vi "svx_Build Orbit and Timebase Data (Unfiltered).vi"(4 "pair index":cluster{"index 1":i32, "index 2":i32}[](array[cluster]), 6 "channel properties":T5[](array[typedef]) {"probe angle [deg]" max=360; "direction" items=["CCW", "CW"]}, 8 "error in (no error)":errorcluster, 9 "interpolated pulse positions[s]":dbl[](array[numeric]) format="%.2f", 10 "even-angle channel info":T1[](array[typedef]) {"channel info"."pregain" format="%.2f"; "channel info"."weighting filter" items=["Linear", "A-weighting", "B-weighting", "C-weighting", "ITU-R 468-4", "Dolby", "CCITT", "C-message", "Wb", "Wc", "Wd", "We", "Wf", "Wh", "Wj", "Wk", "Wm", "AES17 20 kHz lowpass", "AES17 40 kHz lowpass", "AES17 20 kHz highpass", "AES17 40 kHz highpass"]; "channel info"."dB reference" format="%^.1e"; "channel info"."engineering units" items=["custom..."=0, "V"=1, "A"=21, "C"=30, "pC"=31, "s"=32, "-"=29, "Pa"=2, "N"=20, "g"=3, "m/s^2"=4, "m/s"=5, "m"=6, "mm/s"=12, "mm"=13, "micron/s"=14, "micron"=15, "in/s^2"=7, "in/s"=8, "in"=9, "mil/s"=10, "mil"=11, "rad/s^2"=16, "rad/s"=17, "rad"=18, "deg/s^2"=26, "deg/s"=27, "deg"=28, "RPM"=22, "cycle/s^2"=23, "Hz"=24, "cycle"=25, "strain"=19]; "channel info"."sensor sensitivity" format="%#_5f"}, 11 "resampled signal out":cluster{dbl[], dbl}[](array[cluster])) -> (0 "error out":errorcluster, 3 "orbit/timebase plot":T6(array[cluster]))   [LabVIEW 2017]
uses:
  <vilib>/addons/Sound and Vibration/Order Analysis/Data Presentation/SubVIs/OAT MCM Channel Property.ctl
  <vilib>/addons/_NISVFA/_Shared subVIs/Controls/svc_Resampled Channel Info.ctl
  <vilib>/addons/_NISVFA/_Shared subVIs/Controls/svc_Channel Info.ctl
  <vilib>/addons/_NISVFA/_Shared subVIs/Controls/svc_Engineering Units Text Ring.ctl
  <vilib>/addons/_NISVFA/_Shared subVIs/Controls/svc_Weighting Filter Text Ring.ctl
  <vilib>/addons/Sound and Vibration/Order Analysis/Misc/SVMS Attribute.ctl
  <vilib>/addons/_NISVFA/_Shared subVIs/Controls/NI Channel Properties.ctl
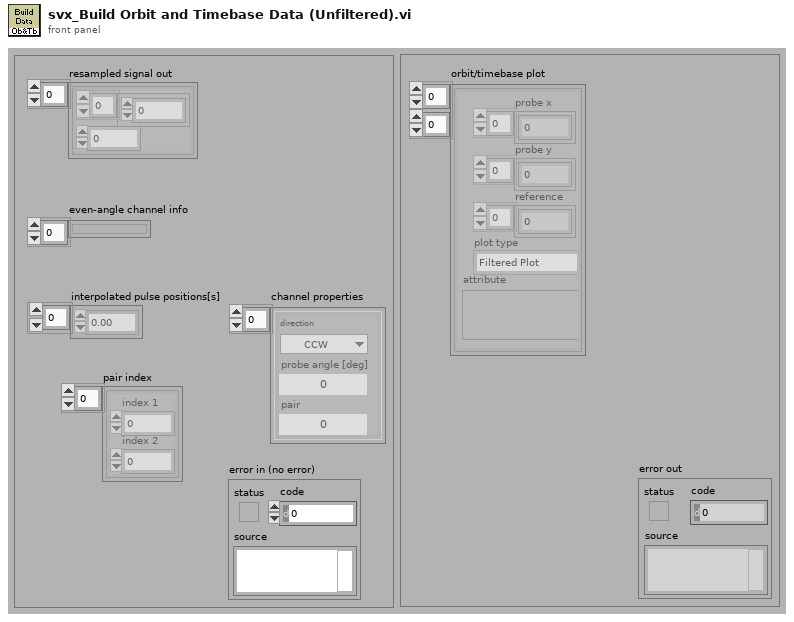
[diagram p1: front panel]
types:
  T1 = typedef "svc_Resampled Channel Info.ctl" = cluster{"channel name":string, "description":string, " channel info":T2}
  T2 = typedef "svc_Channel Info.ctl" = cluster{"sensor sensitivity":dbl, "engineering units":T3, "dB reference":dbl, "custom label":string, "weighting filter":T4, "pregain":dbl}
  T3 = typedef "svc_Engineering Units Text Ring.ctl" = u16
  T4 = typedef "svc_Weighting Filter Text Ring.ctl" = u16
  T5 = typedef "OAT MCM Channel Property.ctl" = cluster{"direction":u16, "probe angle [deg]":u16, "pair":u16}
  T6 = cluster{"probe x":dbl[], "probe y":dbl[], "reference":dbl[], "plot type":enum16{"Filtered Plot", "Unfiltered Plot"}, "attribute":variant}[][]
  T7 = cluster{"X":dbl[], "Y":dbl[], "reference":dbl[], "plot type":enum16{"Filtered Plot", "Unfiltered Plot"}, "attribute":variant}
  T8 = typedef "NI Channel Properties.ctl" = u16
  T9 = typedef "SVMS Attribute.ctl" = u16
  T10 = cluster{"X":dbl[], "Y":dbl[], "reference":dbl[], "plot type":enum16{"Filtered Plot", "Unfiltered Plot"}, "attribute":variant}[]
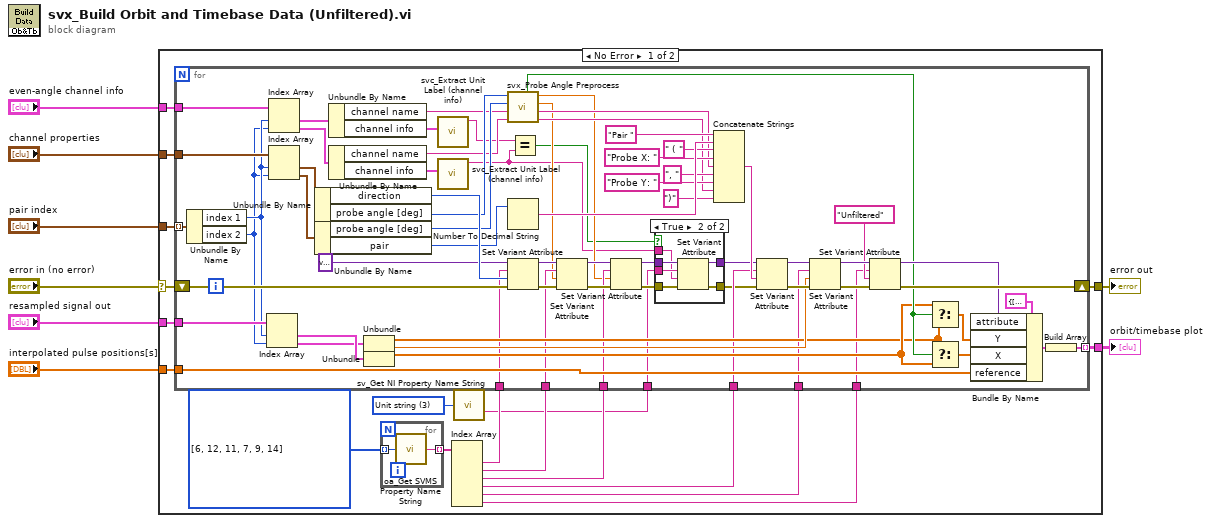
[diagram p0: block diagram]
diagram:
  n1 = case shown="No Error" "error in (no error)" {
    selector: "error in (no error)" -> [w24 w106]
    tunnel: "channel properties" -> [w26 _]
    tunnel: "resampled signal out" -> [w25 _]
    tunnel: [w23 w106] -> w5
    tunnel: [w19 _] -> w1
    tunnel: "interpolated pulse positions[s]" -> [w22 _]
    tunnel: "even-angle channel info" -> [w21 _]
    tunnel: "pair index" -> [w20 _]
    frame No Error {
      w10 = T8 3 items=["Channel name", "Channel description", "Axis label", "Unit string", "Waveform X-axis label", "Waveform X-axis unit string", "x0", "dx", "Number of samples", "X channel", "Filter settled", "dB reference", "Window", "Window parameter", "Window size", "FFT size", "Peak units", "Spectrum type", "Magnitude scale", "Spectral density", "Sensor sensitivity (mV/EU)", "X-axis dimension", "LabVIEW datatype", "Function type", "Function subtype", "X values", "Independent channel", "Column index", "Collection name", "Collection ID", "X Columns", "Phase unwrapped", "Sensor type", "Sensor maximum", "Averaging mode"] ("property")
      w18 = T9[] [6, 12, 11, 7, 9, 14] items=["Pulse / Revolution", "Slope", "Threshold", "Hysteresis", "Order", "Reference Label", "Rotation Direction", "Pair String", "Polar Plot Type", "Sample Per Revolution", "Probe Angle", "Probe Angle X", "Probe Angle Y", "X Axis Unit", "OTB Plot Type"]
      n2 = for {
        tunnel: w18 -> [w28] mode=indexing
        tunnel: [w27] -> w17 mode=indexing
        n3 = call <vilib>:"oa_Get SVMS Property Name String.vi"("attribute"=w28) -> ("attribute name"=w27:string)  [unwired: 4 in]
      }
      n4 = Index Array(array=w17) -> (element #1=w16:string, element #2=w15:string, element #3=w14:string, element #4=w13:string, element #5=w12:string, element #6=w11:string)  [unwired: 6 in]
      n5 = call <vilib>:"sv_Get NI Property Name String.vi"("property"=w10) -> ("WDT attribute name"=w9:string)  [unwired: 13 in, 1 out]
      n6 = for {
        shift-right: [w97] -> w23
        shift-left: w24 -> [w72]
        tunnel: w22 -> [w96]
        tunnel: w20 -> [w71] mode=indexing
        tunnel: w26 -> [w70]
        tunnel: w21 -> [w67]
        tunnel: w25 -> [w66]
        tunnel: [w58] -> w19 mode=indexing
        tunnel: w16 -> [w47]
        tunnel: w15 -> [w46]
        tunnel: w14 -> [w45]
        tunnel: w13 -> [w44]
        tunnel: w12 -> [w43]
        tunnel: w11 -> [w42]
        tunnel: w9 -> [w29]
        n7 = Unbundle By Name(w71) -> ("index 1"=w65:i32, "index 2"=w64:i32)
        n8 = Index Array(array=w66, index #1=w65, index #2=w64) -> (element #1=w61:cluster{dbl[], dbl}, element #2=w60:cluster{dbl[], dbl})
        n9 = Index Array(array=w67, index #1=w65, index #2=w64) -> (element #1=w63:T1, element #2=w62:T1)
        n10 = Index Array(array=w70, index #1=w65, index #2=w64) -> (element #1=w69:T5, element #2=w68:T5)
        n11 = Unbundle By Name(w69) -> ("direction"=w91:u16, "probe angle [deg]"=w57:u16)
        n12 = Unbundle By Name(w68) -> ("probe angle [deg]"=w56:u16, "pair"=w81:u16)
        n13 = Unbundle By Name(w63) -> ("channel name"=w55:string, "channel info"=w40:T2)
        n14 = Unbundle By Name(w62) -> ("channel name"=w54:string, "channel info"=w39:T2)
        n15 = Unbundle(w60) -> (w49:dbl[], w83:dbl)
        n16 = Unbundle(w61) -> (w50:dbl[])  [unwired: 1 out]
        n17 = call <vilib>:"svc_Extract Unit Label (channel info).vi"("channel info"=w40) -> ("unit label"=w36:string)  [unwired: 8 in, 2 out]
        n18 = call <vilib>:"svc_Extract Unit Label (channel info).vi"("channel info"=w39) -> ("unit label"=w30:string)  [unwired: 8 in, 2 out]
        n19 = call <vilib>:"svx_Probe Angle Preprocess.vi"("channel name Y"=w54, "channel name X"=w55, "Y"=w56, "X"=w57) -> ("actual Y"=w41:string, "actual X"=w53:string, "Y"=w38:dbl, "X"=w37:dbl, "switched?"=w51:bool)  [unwired: 3 in]
        n20 = Number To Decimal String(number=w81) -> (decimal integer string=w79:string)  [unwired: 1 in]
        n21 = Set Variant Attribute(Variant=variant ("variant"), name=w47, value=w91, error in=w72) -> (Variant out=w95:variant, error out=w94:errorcluster)  [unwired: 1 out]
        n22 = Equal?(x=w36, y=w30) -> (x = y?=w35:bool)
        n23 = Set Variant Attribute(Variant=w95, name=w46, value=w38, error in=w94) -> (Variant out=w92:variant, error out=w93:errorcluster)  [unwired: 1 out]
        n24 = Set Variant Attribute(Variant=w92, name=w45, value=w37, error in=w93) -> (Variant out=w33:variant, error out=w34:errorcluster)  [unwired: 1 out]
        n25 = case shown="True" w35 {
          tunnel: w34 -> [w98 w105]
          tunnel: w33 -> [w99 w104]
          tunnel: [w98 w103] -> w32
          tunnel: [w99 w102] -> w31
          tunnel: w29 -> [_ w101]
          tunnel: w30 -> [_ w100]
          frame False {
          }
          frame True {
            n26 = Set Variant Attribute(Variant=w104, name=w101, value=w100, error in=w105) -> (Variant out=w102:variant, error out=w103:errorcluster)  [unwired: 1 out]
          }
        }
        n27 = Concatenate Strings("Pair " ("string"), w79, " ( " ("string"), "Probe X: " ("string"), w53, ", " ("string"), "Probe Y: " ("string"), w41, ")" ("string")) -> (w75:string)
        n28 = Set Variant Attribute(Variant=w31, name=w44, value=w75, error in=w32) -> (Variant out=w89:variant, error out=w88:errorcluster)  [unwired: 1 out]
        n29 = Set Variant Attribute(Variant=w89, name=w43, value=w83, error in=w88) -> (Variant out=w86:variant, error out=w87:errorcluster)  [unwired: 1 out]
        n30 = Set Variant Attribute(Variant=w86, name=w42, value="Unfiltered" ("name"), error in=w87) -> (Variant out=w82:variant, error out=w97:errorcluster)  [unwired: 1 out]
        n31 = Select(t=w50, s=w51, f=w49) -> (s? t:f=w52:dbl[])
        n32 = Select(t=w49, s=w51, f=w50) -> (s? t:f=w48:dbl[])
        n33 = Bundle By Name(cluster=T7 {"X"=[], "Y"=[], "reference"=[], "plot type"=enum."Unfiltered Plot", "attribute"=variant} ("orbit plot 2"), "attribute"=w82, "Y"=w52, "X"=w48, "reference"=w96) -> (w59:T7)
        n34 = Build Array(w59) -> (w58:T10)
      }
    }
    frame Error {
    }
  }
  "orbit/timebase plot" <- w1
  "error out" <- w5
